vi "modify channel test.vi"() -> ()   [LabVIEW 2013, in "sample module tests.lvlib"]
uses:
  sample module tests.lvlib
  channel/TBM channel.lvclass/TBM channel.ctl
  channel/channel classification.ctl
  module/configuration/sample module configuration.lvclass
  <vilib>/NI/Tag Bus/tag/tag descriptor.lvclass/tag descriptor.ctl
  channel/Read channel classification.vi
  channel/Write channel classification.vi
  <vilib>/NI/Tag Bus/tag/read tag name.vi
  channel/TBM channel.lvclass
panel:
  out "rename success":bool
  out "no err":errorcluster
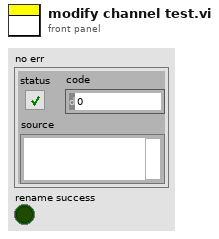
[diagram p1: front panel]
types:
  T1 = typedef "TBM channel.lvclass/channel classification.ctl" = enum16{"input data", "output data", "processing parameter", "processing result"}
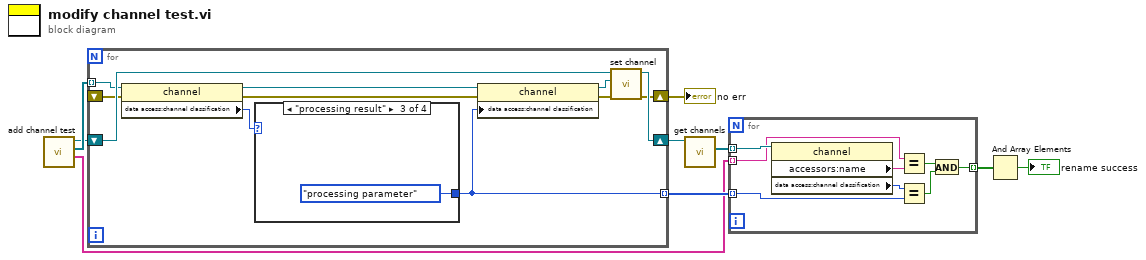
[diagram p0: block diagram]
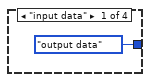
[diagram p2: hidden frame]
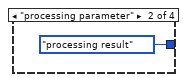
[diagram p3: hidden frame]
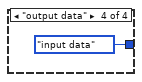
[diagram p4: hidden frame]
diagram:
  n1 = call "add channel test.vi"() -> ("names"=w3:string[], "channels"=w2:refnum<class "TBM channel.lvclass">[], "sample module configuration out"=w1:refnum<class "sample module configuration.lvclass">)  [unwired: 8 in, 1 out]
  n2 = for {
    shift-right: [w19] -> w9
    shift-left: w1 -> [w20]
    shift-right: [w18] -> w8
    shift-left: _ -> [w17]
    tunnel: w2 -> [w15] mode=indexing
    tunnel: [w10] -> w4 mode=indexing
    n3 = property class="channel"(reference=w15, error in=w17) -> (reference out=w13:refnum<class "TBM channel.lvclass">, error out=w16:errorcluster, "data access:channel classification"=w11:T1)
    n4 = case shown="\"processing result\"" w11 {
      tunnel: [channel_classification."output data" ("channel classification") channel_classification."processing result" ("channel classification") channel_classification."processing parameter" ("channel classification") channel_classification."input data" ("channel classification")] -> w10
      frame "input data" {
      }
      frame "processing parameter" {
      }
      frame "processing result" {
      }
      frame "output data" {
      }
    }
    n5 = property class="channel"(reference=w13, error in=w16, "data access:channel classification"=w10) -> (reference out=w12:refnum<class "TBM channel.lvclass">, error out=w14:errorcluster)
    n6 = call "set channel.vi"("error in"=w14, "channel"=w12, "sample module configuration in"=w20) -> ("error out"=w18:errorcluster, "sample module configuration out"=w19:refnum<class "sample module configuration.lvclass">)  [unwired: 7 in]
  }
  "no err" <- w8
  n7 = call-dynamic "get channels.vi"("module configuration in"=w9) -> ("channels"=w7:refnum<class "TBM channel.lvclass">[])  [unwired: 9 in, 1 out]
  n8 = for {
    tunnel: w7 -> [w31] mode=indexing
    tunnel: [w30] -> w6 mode=indexing
    tunnel: w4 -> [w29] mode=indexing
    tunnel: w3 -> [w26] mode=indexing
    n9 = property class="channel"(reference=w31) -> ("accessors:name"=w27:string, "data access:channel classification"=w28:T1)  [unwired: 1 in, 2 out]
    n10 = Equal?(x=w26, y=w27) -> (x = y?=w25:bool)
    n11 = Equal?(x=w28, y=w29) -> (x = y?=w32:bool)
    n12 = And(x=w25, y=w32) -> (x .and. y?=w30:bool)
  }
  n13 = And Array Elements(Boolean array=w6) -> (logical AND=→"rename success":bool)
